vi "INIT TGM.vi"(8 "error in (no error)":errorcluster, 11 "QPA Measurement in":refnum<class "QPA Measurement.lvclass">) -> (0 "error out":errorcluster, 3 "QPA Measurement out":refnum<class "QPA Measurement.lvclass">)   [LabVIEW 2016, in "QPA Measurement.lvlib" / "QPA Measurement.lvclass"]
uses:
  QPA Measurement.lvclass
  Plugins/Test Group Manager.lvlibp/Test Group Manager.lvclass
  QPA Measurement.lvclass/QPA Measurement.ctl
  Protected Methods/Write Test Group Manager.vi
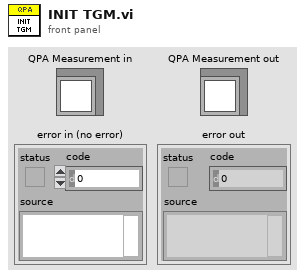
[diagram p1: front panel]
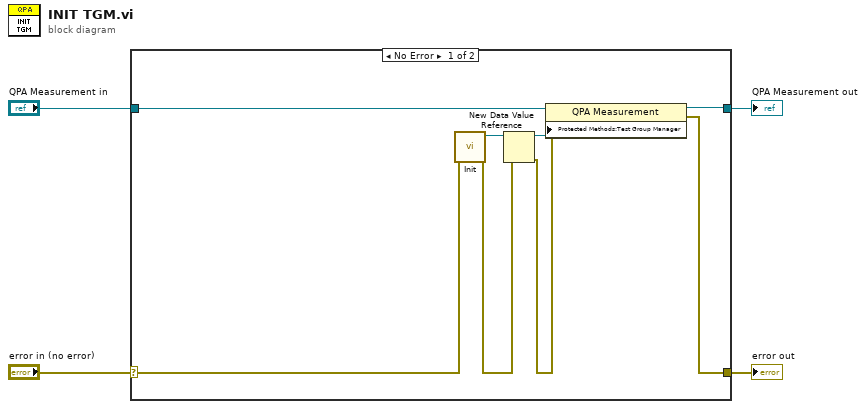
[diagram p0: block diagram]
diagram:
  n1 = case shown="No Error" "error in (no error)" {
    selector: "error in (no error)" -> [w9 w14]
    tunnel: [w12 w14] -> w3
    tunnel: [w10 w13] -> w1
    tunnel: "QPA Measurement in" -> [w11 w13]
    frame No Error {
      n2 = call "Init.vi"("error in (no error)"=w9) -> ("error out"=w6:errorcluster, "Test Group Manager out"=w8:refnum<class "Test Group Manager.lvclass">)  [unwired: 9 in]
      n3 = New Data Value Reference(data value=w8, error in=w6) -> (data value reference=w7:refnum<data-value>, error out=w5:errorcluster)
      n4 = property class="QPA Measurement"(reference=w11, error in=w5, "Protected Methods:Test Group Manager"=w7) -> (reference out=w10:refnum<class "QPA Measurement.lvclass">, error out=w12:errorcluster)
    }
    frame Error {
    }
  }
  "error out" <- w3
  "QPA Measurement out" <- w1
